vi "Delete Waveform.vi"(8 "error in (no error)":errorcluster, 10 "Waveform.lvclass":refnum<class "Waveform.lvclass">, 11 "Composite Waveform in":refnum<class "Composite Waveform.lvclass">) -> (0 "error out":errorcluster, 3 "Composite Waveform out":refnum<class "Composite Waveform.lvclass">)   [LabVIEW 2014, in "Composite Waveform.lvclass"]
uses:
  Composite Waveform.lvclass
  Waveform/Waveform.lvclass
panel:
  in  "Waveform Index":i32
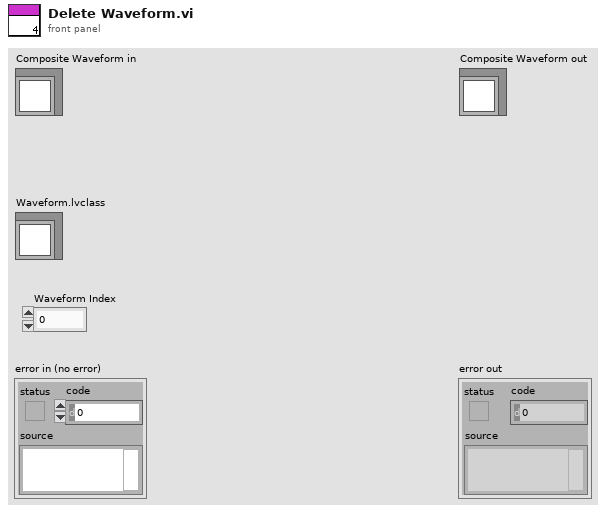
[diagram p1: front panel]
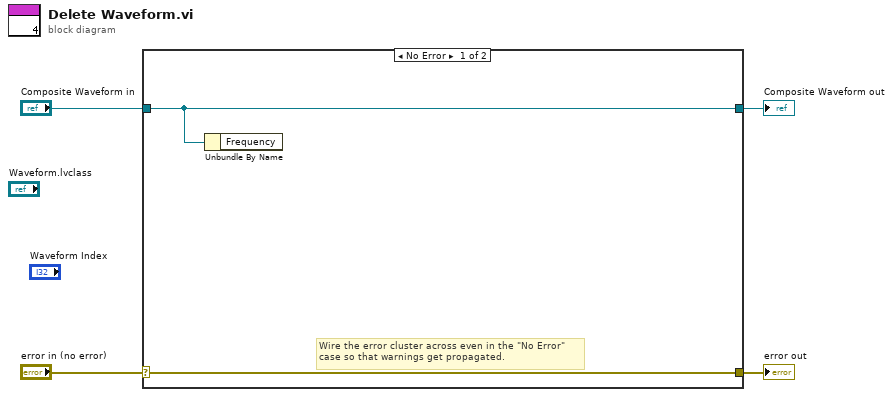
[diagram p0: block diagram]
diagram:
  n1 = case shown="No Error" "error in (no error)" {
    selector: "error in (no error)" -> [w6 w8]
    tunnel: [w6 w8] -> w3
    tunnel: [w5 w7] -> w1
    tunnel: "Composite Waveform in" -> [w5 w7]
    frame No Error {
      # "Wire the error cluster across even in the \"No Error\"\ncase so that warnings get propagated."
      n2 = Unbundle By Name(w5) -> ()  [unwired: 1 out]
    }
    frame Error {
    }
  }
  "error out" <- w3
  "Composite Waveform out" <- w1
